vi "Watch_Current.vi"() -> ()   [LabVIEW 2023]
uses:
  Sub_Vi/TypeDefsControls/Voltage.ctl
  Sub_Vi/TypeDefs/WayPointCluster.ctl
  Sub_Vi/TypeDefs/Settings.ctl
  Sub_Vi/TypeDefs/ChangeOnFly.ctl
  Sub_Vi/TypeDefs/Display.ctl
  Settings.vi
panel:
  in  "stop":bool
  in  "SaveData?":bool
  in  "AO4 Voltage (V)":T1 min=-10.0 max=10.0
  in  "AO3 Voltage (V)":T1 min=-10.0 max=10.0
  in  "Display Cluster":T2
  in  "ChangeonFly":T3
  in  "SettingsCluster":T4={"Sample Rate (us)"=1, "Samples Per Data Point (int, power of 2)"=1000, "DistanceToBulk (um)"=-1.0, "HoldTimeScaler"=1, "SaveData"=TRUE, "DistanceToBulk (um) 2"=-1.0, "DistanceToBulk (um) 3"=-1.0}
  in  "WayPointCluster":T5
  in  "Tab Control":enum32{"Current Followers", "Piezos"}(tab)
  out "t vs Current 2":dbl[](graph)
  out "t vs Current 3":dbl[](graph)
  out "t vs Current 1":dbl[](graph)
  out "t vs Z Position":dbl[](graph)
  out "t vs Y Position":dbl[](graph)
  out "t vs X Position":dbl[](graph)
  # "Controls"
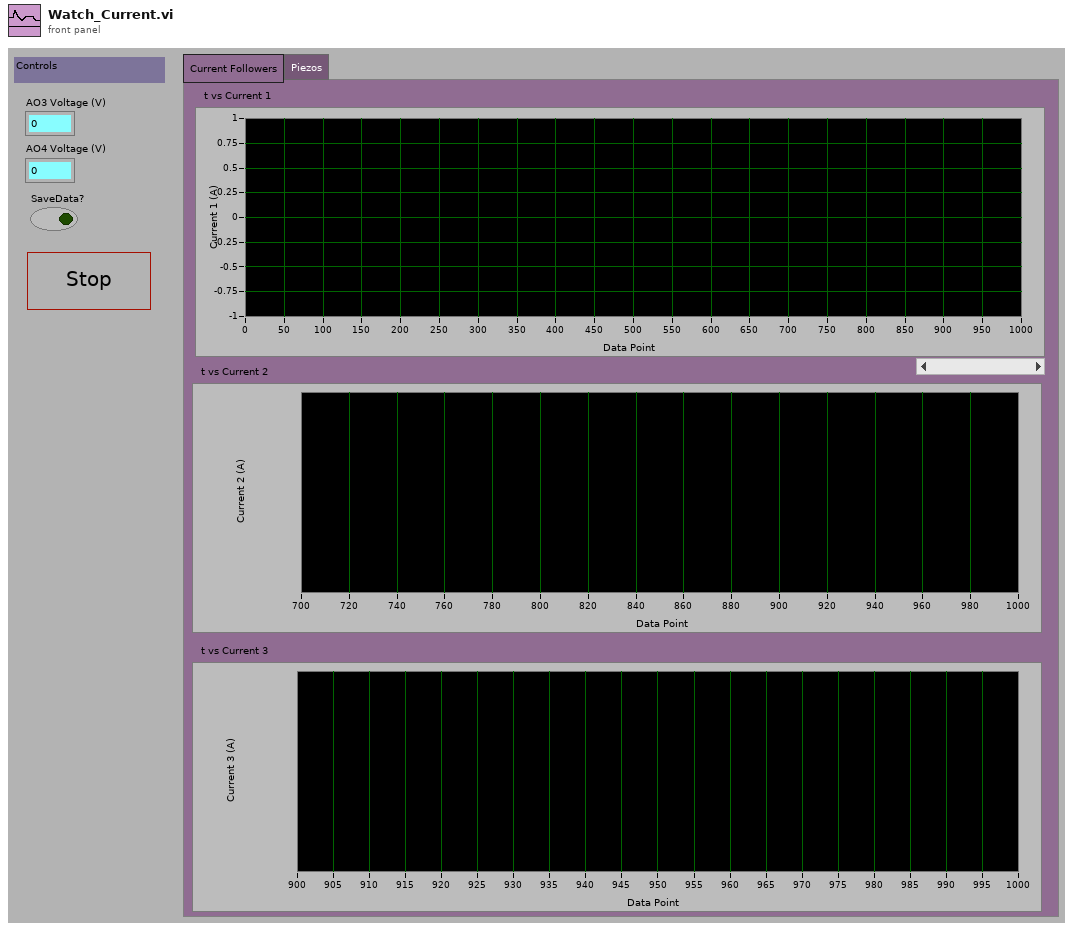
[diagram p1: front panel]
types:
  T1 = typedef "Voltage.ctl" = dbl
  T2 = typedef "Display.ctl" = cluster{"X":refnum<vi>, "Y":refnum<vi>, "Z":refnum<vi>, "Amp":refnum<vi>, "Phase":refnum<vi>, "t vs Z":refnum<vi>, "t vs C1":refnum<vi>, "t vs C2":refnum<vi>, "t vs C3":refnum<vi>, "t vs Amp":refnum<vi>, "t vs Phase":refnum<vi>, "t vs X":refnum<vi>, "t vs Y":refnum<vi>, "Z vs C1":refnum<vi>, "Z vs C2":refnum<vi>, "Z vs C3":refnum<vi>, "V vs C1":refnum<vi>, "V vs C2":refnum<vi>, "V vs C3":refnum<vi>, "X/Y/Z F":refnum<vi>, "X/Y/Z R":refnum<vi>, "X/Y/C1 F":refnum<vi>, "X/Y/C1 R":refnum<vi>, "X/Y/C2 F":refnum<vi>, "X/Y/C2 R":refnum<vi>, "X/Y/C3 F":refnum<vi>, "X/Y/C3 R":refnum<vi>, "NumberOfLines":u16, "um Per Pixel":dbl, "um Per Line":dbl, "X Center":dbl, "Hop X/Y/Z":refnum<vi>, "Hop X/Y/C1":refnum<vi>, "Hop X/Y/C2":refnum<vi>, "Hop X/Y/C3":refnum<vi>, "X Width":dbl, "Y Width":dbl, "Hopping Distance":dbl, "V2 vs C1":refnum<vi>, "V vs Phase":refnum<vi>, "Y Center":dbl, "Number of Pixels":dbl, "V2 vs C2":refnum<vi>, "V2 vs C3":refnum<vi>, "V vs y":refnum<vi>, "V2 vs y":refnum<vi>, "Z vs Amp":refnum<vi>, "Z vs Phase":refnum<vi>}
  T3 = typedef "ChangeOnFly.ctl" = cluster{"Stop (boolean)":refnum<vi>, "Pause (boolean)":refnum<vi>, "EndCurrentLine (boolean)":refnum<vi>, "max movement per update step (Interger, nm)":refnum<vi>, "P (float, arb)":refnum<vi>, "Feedback set point (double, Amps)":refnum<vi>, "Voltage (double, V)":refnum<vi>, "Feedback set point 2 (double, Amps)":refnum<vi>, "Stop on Greater Than 2? (boolean)":refnum<vi>, "Stop on Greater Than? (boolean)":refnum<vi>, "Voltage 2 (double, V)":refnum<vi>, "Feedback Type (enum)":refnum<vi>, "Feedback Type 2 (enum)":refnum<vi>}
  T4 = typedef "Settings.ctl" = cluster{"Sample Rate (us)":u32, "Samples Per Data Point (int, power of 2)":i16, "DistanceToBulk (um)":dbl, "HoldTimeScaler":u64, "SaveData":bool, "DistanceToBulk (um) 2":dbl, "DistanceToBulk (um) 3":dbl}
  T5 = typedef "WayPointCluster.ctl" = cluster{"X (um)":dbl[], "Y (um)":dbl[], "Z (um)":dbl[], "V (V)":dbl[], "X Velocity (um s-1)":dbl[], "Y Velocity (um s-1)":dbl[], "Z Velocity (um s-1)":dbl[], "V Velocity (V s-1)":dbl[], "FeedBack Type (enum)":u16[], "Move X (boolean)":bool[], "Move Y (boolean)":bool[], "Move Z (boolean)":bool[], "Move V (boolean)":bool[], "Jump V (boolean)":bool[], "Hold (boolean)":bool[], "Hold Time":u32[], "V2 (V)":dbl[], "Move V2":bool[], "V2 Velocity (V s-1)":dbl[], "Jump V2 (boolean)":bool[], "Update z Position delta (ms)":i16[], "Hold Feedback1":bool[], "Move Z PicoMotor":bool[], " Z PicoMotor Direction":bool[], "DIO0":bool[]}
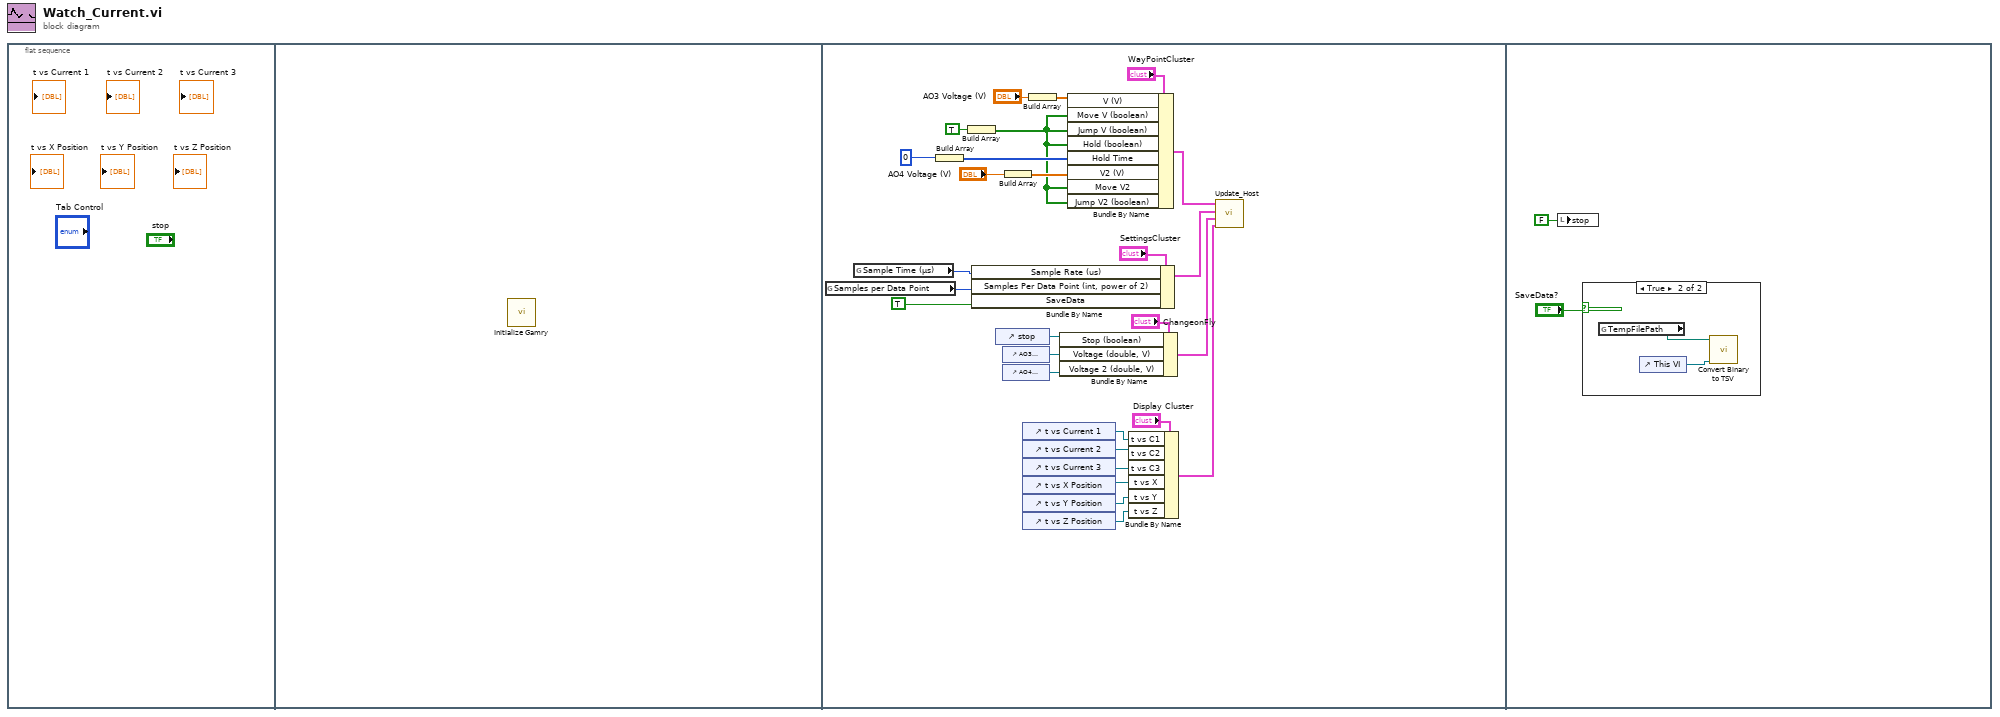
[diagram p0: block diagram]
diagram:
  n1 = flat-sequence {
    frame #0 {
    }
    frame #1 {
      n2 = call "Initialize Gamry.vi"() -> ()  [unwired: 12 in]
    }
    frame #2 {
      n3 = global read "Settings.vi" "Samples per Data Point"() -> (w17:u16)
      n4 = global read "Settings.vi" "Sample Time (µs)"() -> (w16:u32)
      n5 = Build Array(i16 0 ("y")) -> (w22:i16[])
      n6 = Build Array(TRUE ("Change V on Fly")) -> (w13:bool[])
      n7 = Bundle By Name(cluster="SettingsCluster", "Sample Rate (us)"=w16, "Samples Per Data Point (int, power of 2)"=w17, "SaveData"=TRUE) -> (w11:T4)
      n8 = control-ref of="stop"() -> (w3:refnum<vi>)
      n9 = control-ref of="AO3 Voltage (V)"() -> (w4:refnum<vi>)
      n10 = control-ref of="AO4 Voltage (V)"() -> (w2:refnum<vi>)
      n11 = Build Array("AO4 Voltage (V)") -> (w14:T1[])
      n12 = control-ref of="t vs Current 1"() -> (w8:refnum<vi>)
      n13 = control-ref of="t vs Current 2"() -> (w7:refnum<vi>)
      n14 = control-ref of="t vs Current 3"() -> (w26:refnum<vi>)
      n15 = control-ref of="t vs X Position"() -> (w25:refnum<vi>)
      n16 = control-ref of="t vs Y Position"() -> (w6:refnum<vi>)
      n17 = control-ref of="t vs Z Position"() -> (w5:refnum<vi>)
      n18 = Build Array("AO3 Voltage (V)") -> (w27:T1[])
      n19 = Bundle By Name(cluster="ChangeonFly", "Stop (boolean)"=w3, "Voltage (double, V)"=w4, "Voltage 2 (double, V)"=w2) -> (w9:T3)
      n20 = Bundle By Name(cluster="WayPointCluster", "V (V)"=w27, "Move V (boolean)"=w13, "Jump V (boolean)"=w13, "Hold (boolean)"=w13, "Hold Time"=w22, "V2 (V)"=w14, "Move V2"=w13, "Jump V2 (boolean)"=w13) -> (w12:T5)
      n21 = Bundle By Name(cluster="Display Cluster", "t vs C1"=w8, "t vs C2"=w7, "t vs C3"=w26, "t vs X"=w25, "t vs Y"=w6, "t vs Z"=w5) -> (w10:T2)
      n22 = call "Update_Host.vi"("Display Cluster"=w10, "ChangeonFly"=w9, "SettingsCluster"=w11, "WayPointCluster"=w12) -> ()  [unwired: 6 in]
    }
    frame #3 {
      n23 = local write "stop"(FALSE ("stop")) -> ()
      n24 = case shown="True" "SaveData?" {
        frame False {
        }
        frame True {
          n25 = global read "Settings.vi" "TempFilePath"() -> (w31:path)
          n26 = control-ref of="This VI"() -> (w32:refnum<vi>)
          n27 = call "Convert Binary to TSV.vi"("This VI"=w32, "TDMS DataFile Name"=w31) -> ()  [unwired: 10 in]
        }
      }
    }
  }
